vi "DAQ_create_shutters_arrays.vi"(2 "error in":errorcluster, 3 "Channel Names In":string[](array[string]), 4 "new task name":string, 5 "Lines in":string[](array[string])) -> (0 "error out":errorcluster, 1 "task out":refnum<k21>)   [LabVIEW 2015]
uses:
  <vilib>/DAQmx/create/channels.llb/DAQmx Create Channel (DO-Digital Output).vi
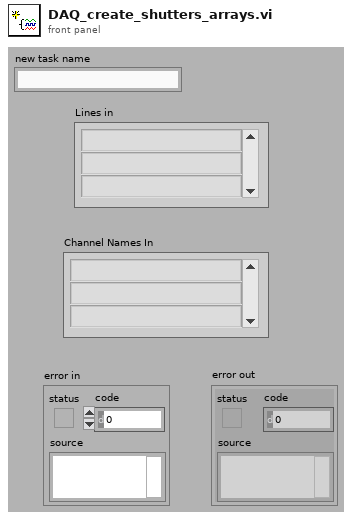
[diagram p1: front panel]
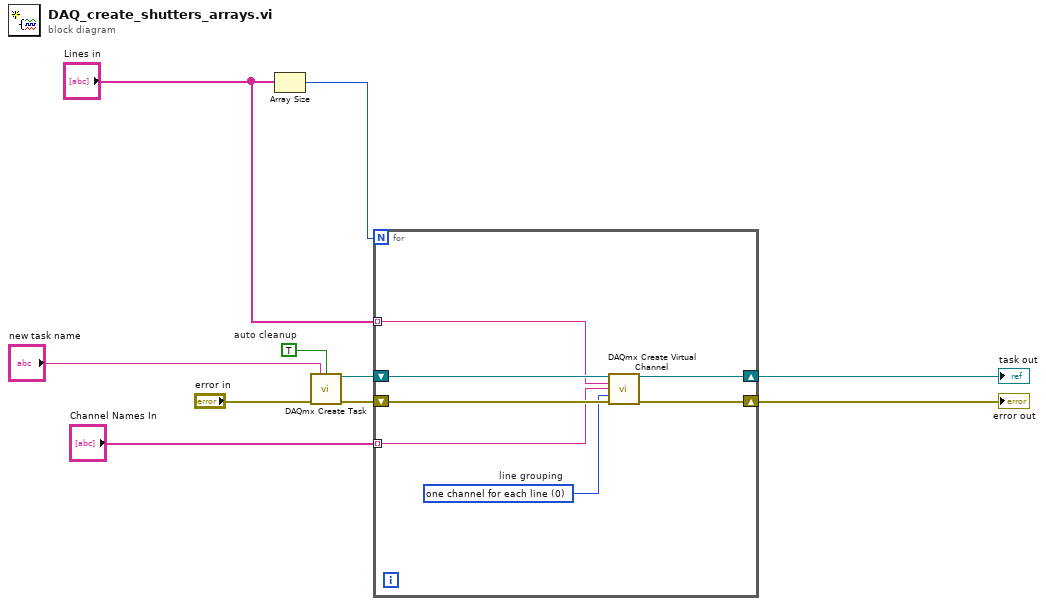
[diagram p0: block diagram]
diagram:
  w8 = TRUE  # auto cleanup
  n1 = Array Size(array="Lines in") -> (size(s)=w4:i32)
  n2 = call <vilib>:"DAQmx Create Task.vi"("new task name"="new task name", "auto cleanup"=w8, "error in"="error in") -> ("task out"=w7:refnum<k21>, "error out"=w9:errorcluster)  [unwired: 11 in]
  n3 = for {
    N: w4 -> [_]
    shift-right: [w13] -> w5
    shift-left: w9 -> [w17]
    shift-right: [w14] -> w6
    shift-left: w7 -> [w16]
    tunnel: "Lines in" -> [w12] mode=indexing
    tunnel: "Channel Names In" -> [w11] mode=indexing
    w15 = 0 items=["one channel for each line", "one channel for all lines"]  # line grouping
    n4 = call-poly <vilib>:"DAQmx Create Virtual Channel.vi"("task in"=w16, "lines"=w12, "name to assign"=w11, "line grouping"=w15, "error in"=w17) -> ("task out"=w14:refnum<k21>, "error out"=w13:errorcluster)  [unwired: 9 in]
  }
  "error out" <- w5
  "task out" <- w6
